vi "Ev Cmd Write Configuration.vi"(8 "error in (no error)":errorcluster, 10 "Configuration":T1={"Language"={"Name"=""}, "Path Config"={"Data Folder Path"=path "", "PNG Folder Path"=path "", "mp3 Folder Path"=path ""}, "Image Viewer Config"={"Center Point"={"Size"=3, "Color"=0, "Show?"=FALSE}, "bp Point"={"Size"=3, "Color"=0, "Show?"=FALSE}, "w Point"={"Size"=3, "Color"=0, "Show?"=FALSE}, "b Box"={"Fill Color"=0, "Border Color"=0, "Show?"=FALSE}, "i Box"={"Fill Color"=0, "Border Color"=0, "Show?"=FALSE}, "o Point"={"Size"=3, "Color"=0, "Show?"=FALSE}, "c Point"={"Size"=3, "Color"=0, "Show?"=FALSE}}}, 11 "LF2R IDE in":refnum<class "Main Panel.lvclass">) -> (0 "error out":errorcluster, 3 "LF2R IDE out":refnum<class "Main Panel.lvclass">)   [LabVIEW 2018, in "Main Panel.lvlib" / "Main Panel.lvclass"]
uses:
  Main Panel.lvclass
  Const Configuration.ctl
  Const Path Setting.ctl
  Const Image Viewer Setting.ctl
  Main Panel.lvclass/Main Panel.ctl
  Framework/Framework/Framework.lvclass
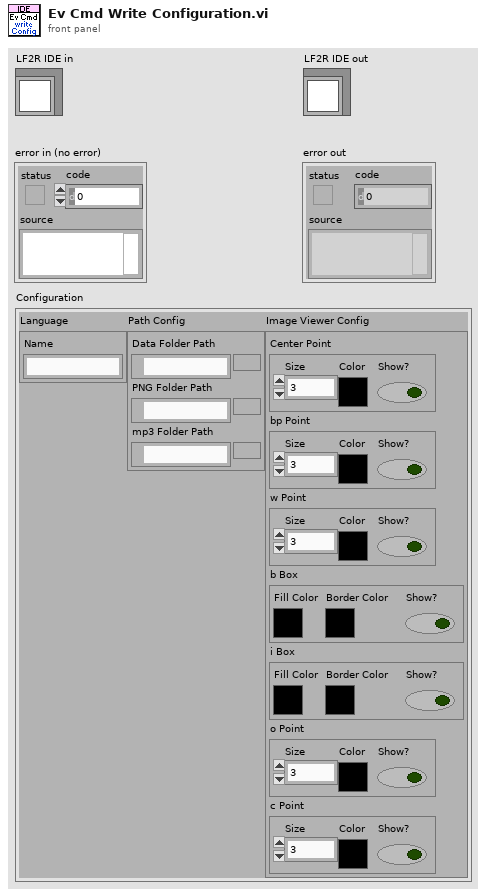
[diagram p1: front panel]
types:
  T1 = typedef "Main Panel.lvlib/Main Panel.lvclass/Const Configuration.ctl" = cluster{"Language":cluster{"Name":string}, "Path Config":T2, "Image Viewer Config":T3}
  T2 = typedef "Main Panel.lvlib/Main Panel.lvclass/Const Path Setting.ctl" = cluster{"Data Folder Path":path, "PNG Folder Path":path, "mp3 Folder Path":path}
  T3 = typedef "Main Panel.lvlib/Main Panel.lvclass/Const Image Viewer Setting.ctl" = cluster{"Center Point":cluster{"Size":i32, "Color":u32, "Show?":bool}, "bp Point":cluster{"Size":i32, "Color":u32, "Show?":bool}, "w Point":cluster{"Size":i32, "Color":u32, "Show?":bool}, "b Box":cluster{"Fill Color":u32, "Border Color":u32, "Show?":bool}, "i Box":cluster{"Fill Color":u32, "Border Color":u32, "Show?":bool}, "o Point":cluster{"Size":i32, "Color":u32, "Show?":bool}, "c Point":cluster{"Size":i32, "Color":u32, "Show?":bool}}
  T4 = typedef "Framework.lvlib/Framework.lvclass/Const Lang Setting.ctl" = cluster{"Main Panel":T5, "Configuration Window":T18}
  T5 = typedef "Framework.lvlib/Framework.lvclass/Const Lang MainWnd.ctl" = cluster{"Title":T6, "Frame Basic":T8, "Frame Skill":T9, "bp":T10, "w":T11, "b":T12, "i":T13, "o":T14, "c":T15, "Other":T16, "Menu":T17}
  T6 = typedef "Framework.lvlib/Framework.lvclass/Const Lang MainWnd Frame Title.ctl" = cluster{"Frame Num":T7, "Name":T7}
  T7 = typedef "Framework.lvlib/Framework.lvclass/Const Lang Property.ctl" = cluster{"Name":string, "Tip":string, "Description":string}
  T8 = typedef "Framework.lvlib/Framework.lvclass/Const Lang MainWnd Frame Basic.ctl" = cluster{"pic":T7, "state":T7, "wait":T7, "next":T7, "dvx":T7, "dvy":T7, "dvz":T7, "centerx":T7, "centery":T7, "sound":T7}
  T9 = typedef "Framework.lvlib/Framework.lvclass/Const Lang MainWnd Frame Skill.ctl" = cluster{"mp":T7, "hit_a":T7, "hit_d":T7, "hit_j":T7, "hit_Fa":T7, "hit_Ua":T7, "hit_Da":T7, "hit_Fj":T7, "hit_Uj":T7, "hit_Dj":T7, "hit_ja":T7}
  T10 = typedef "Framework.lvlib/Framework.lvclass/Const Lang MainWnd Frame bp.ctl" = cluster{"x":T7, "y":T7}
  T11 = typedef "Framework.lvlib/Framework.lvclass/Const Lang MainWnd Frame w.ctl" = cluster{"kind":T7, "x":T7, "y":T7, "weaponact":T7, "cover":T7, "dvx":T7, "dvy":T7, "dvz":T7, "attacking":T7}
  T12 = typedef "Framework.lvlib/Framework.lvclass/Const Lang MainWnd Frame b.ctl" = cluster{"kind":T7, "x":T7, "y":T7, "w":T7, "h":T7, "index":T7}
  T13 = typedef "Framework.lvlib/Framework.lvclass/Const Lang MainWnd Frame i.ctl" = cluster{"kind":T7, "x":T7, "y":T7, "w":T7, "h":T7, "zwidth":T7, "dvx":T7, "dvy":T7, "dvz":T7, "fall":T7, "arest":T7, "vrest":T7, "bdefend":T7, "injury":T7, "effect":T7, "catchingact 1":T7, "catchingact 2":T7, "caughtact 1":T7, "caughtact 2":T7, "index":T7}
  T14 = typedef "Framework.lvlib/Framework.lvclass/Const Lang MainWnd Frame o.ctl" = cluster{"kind":T7, "x":T7, "y":T7, "action":T7, "dvx":T7, "dvy":T7, "dvz":T7, "oid":T7, "facing":T7}
  T15 = typedef "Framework.lvlib/Framework.lvclass/Const Lang MainWnd Frame c.ctl" = cluster{"kind":T7, "x":T7, "y":T7, "injury":T7, "cover":T7, "vaction":T7, "aaction":T7, "taction":T7, "hurtable":T7, "decrease":T7, "fronthurtact":T7, "backhurtact":T7, "throwvx":T7, "throwvy":T7, "throwvz":T7, "throwinjury":T7, "dircontrol":T7}
  T16 = typedef "Framework.lvlib/Framework.lvclass/Const Lang MainWnd Other.ctl" = cluster{"File Path":T7, "GoTo":T7, "Apply Change":T7, "To Next Frame":T7, "Sound Play":T7}
  T17 = typedef "Framework.lvlib/Framework.lvclass/Const Lang MainWnd Menu.ctl" = cluster{"File":T7, "Open File":T7, "Save File":T7, "Exit":T7, "Settings":T7, "Preferences":T7, "Help":T7, "Show Context Help":T7}
  T18 = typedef "Framework.lvlib/Framework.lvclass/Const Lang CfgWnd.ctl" = cluster{"Tab":T19, "Main":T20, "Path":T21, "Image":T22}
  T19 = typedef "Framework.lvlib/Framework.lvclass/Const Lang CfgWnd Tab.ctl" = cluster{"Main Page":T7, "Image Page":T7}
  T20 = typedef "Framework.lvlib/Framework.lvclass/Const Lang CfgWnd Main.ctl" = cluster{"Language":T7, "Save":T7, "Cancel":T7}
  T21 = typedef "Framework.lvlib/Framework.lvclass/Const Lang CfgWnd Path.ctl" = cluster{"Reset":T7, "Path Data":T7, "Path Png":T7, "Path Mp3":T7}
  T22 = typedef "Framework.lvlib/Framework.lvclass/Const Lang CfgWnd Image.ctl" = cluster{"Center Point":cluster{"Name":T7, "Size":T7, "Color":T7, "Enable":T7}, "bp Point":cluster{"Name":T7, "Size":T7, "Color":T7, "Enable":T7}, "w Point":cluster{"Name":T7, "Size":T7, "Color":T7, "Enable":T7}, "b Box":cluster{"Name":T7, "Fill Color":T7, "Border Color":T7, "Enable":T7}, "i Box":cluster{"Name":T7, "Fill Color":T7, "Border Color":T7, "Enable":T7}, "o Point":cluster{"Name":T7, "Size":T7, "Color":T7, "Enable":T7}, "c Point":cluster{"Name":T7, "Size":T7, "Color":T7, "Enable":T7}}
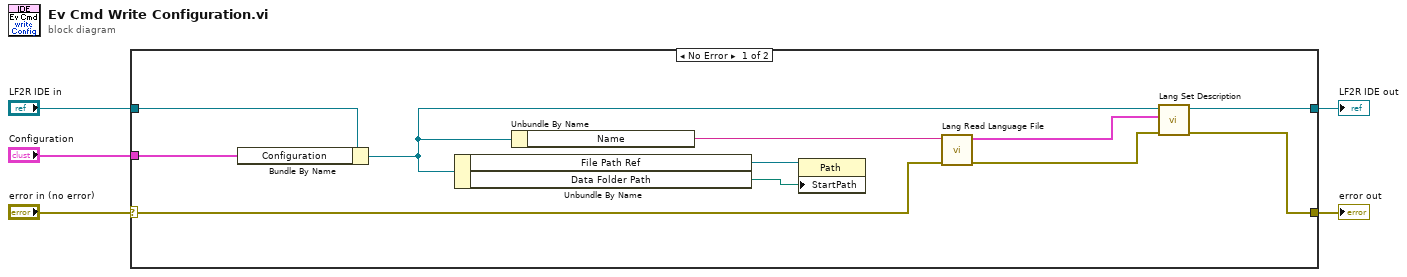
[diagram p0: block diagram]
diagram:
  n1 = case shown="No Error" "error in (no error)" {
    selector: "error in (no error)" -> [w11 w18]
    tunnel: [w10 w18] -> w4
    tunnel: [w9 w17] -> w2
    tunnel: "LF2R IDE in" -> [w16 w17]
    tunnel: "Configuration" -> [w15 _]
    frame No Error {
      n2 = Bundle By Name(cluster=w16, "Configuration"=w15) -> (w8:refnum<class "Main Panel.lvclass">)
      n3 = Unbundle By Name(w8) -> ("File Path Ref"=w14:refnum<vi>, "Data Folder Path"=w13:path)
      n4 = Unbundle By Name(w8) -> ("Name"=w7:string)
      n5 = property class="Path"(reference=w14, "StartPath"=w13) -> ()  [unwired: 1 in, 2 out]
      n6 = call "Lang Read Language File.vi"("error in (no error)"=w11, "Language Name"=w7) -> ("error out"=w12:errorcluster, "UI Descriptions"=w6:T4)  [unwired: 7 in, 1 out]
      n7 = call "Lang Set Description.vi"("error in (no error)"=w12, "UI Descriptions"=w6, "LF2R IDE in"=w8) -> ("error out"=w10:errorcluster, "LF2R IDE out"=w9:refnum<class "Main Panel.lvclass">)  [unwired: 7 in]
    }
    frame Error {
    }
  }
  "error out" <- w4
  "LF2R IDE out" <- w2
